vi "main_FP.vi"() -> ()   [LabVIEW 2011]
uses:
  global.vi
  <vilib>/Instr/_visa.llb/VISA Configure Serial Port (Instr).vi
panel:
  out "RN2483 Connected":bool caption="Connected"
  in  "Tab Control 2":T1(tab)
  out "Receiving":bool
  out "Signal Noise Ratio":string="0"
  out "Packet number":i32
  in  "Stop_reception":bool
  in  "Start_reception":bool
  in  "reception_list":i32(listbox)
  out "reception Graph":dbl[](graph)
  out "Transmitting":bool
  in  "delay (ms)":u32=2000 max=65535 step=1
  in  "tx_timestamp":bool caption="Add timestamp"
  in  "tx_packetnum":bool caption="Add packet number"
  in  "Message":string="0"
  out "TX Packet number":i32 caption="Packet number"
  in  "Stop_transmission":bool
  in  "Start_transmission":bool caption="Start_reception"
  in  "transmission_list":i32(listbox)
  in  "Bandwidth":string(combo)="125"
  in  "CRC":bool
  in  "Preamble length":u32=8 max=65535 step=1
  in  "Frequency":u32=57600 max=65535 step=1
  in  "Bitrate":u32=50000 max=65535 step=1
  in  "Freq deviation":u32=57600 max=65535 step=1
  in  "RX signal bw":string(combo)
  in  "Freq correct":string(combo)
  in  "Spreading factor":string(combo)
  in  "Power":string(combo)
  in  "Radio mode":string(combo)
  out "EUI address":string="\r\n"
  out "Voltage":string="\r\n"
  out "Version":string="0004A30B001A5EB1\r\n"
  in  "Save_changes":bool
  in  "Cancel_changes":bool
  out "error":bool
  in  "Discover device":bool=TRUE
  in  "Timeout (ms)":u32=10000
  in  "Port":refnum<visa-resource-name>="COM1"
  in  "Parity":u16(ring) items=["None", "Odd", "Even", "Mark", "Space"]
  in  "Stop bits":u16(ring)=10 items=["1.0"=10, "1.5"=15, "2.0"=20]
  in  "Baud rate":u32=57600
  in  "Data bits":u16=8
  # "Reception mode"
  # "Transmission mode"
  # "Device info"
  # "Device config"
  # "Serial port"
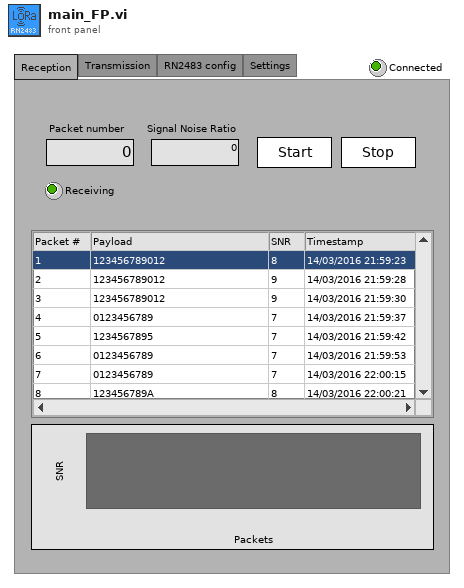
[diagram p1: front panel]
types:
  T1 = enum32{"Reception", "Transmission", "RN2483 config", "Settings"}
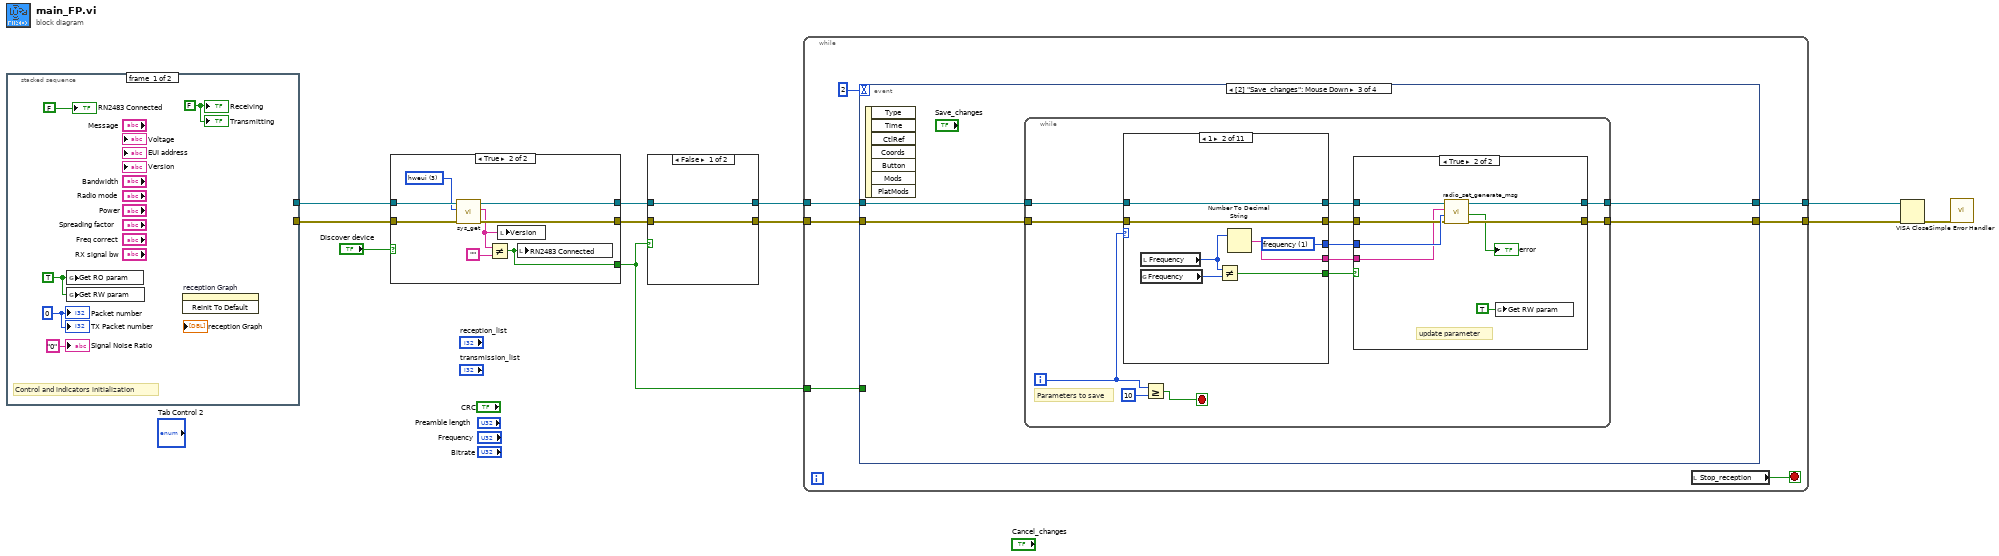
[diagram p0: block diagram]
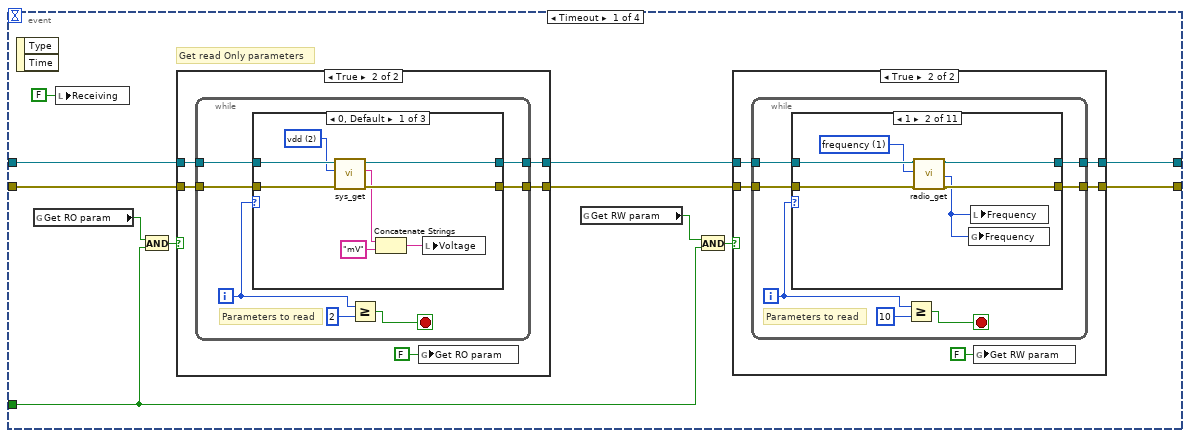
[diagram p2: hidden frame]
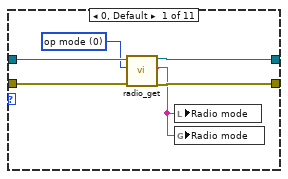
[diagram p4: hidden frame]
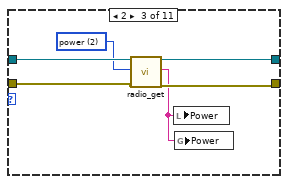
[diagram p5: hidden frame]
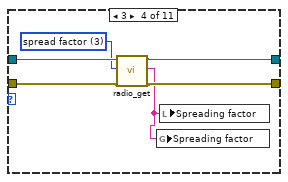
[diagram p6: hidden frame]
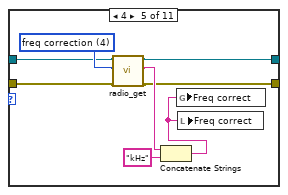
[diagram p7: hidden frame]
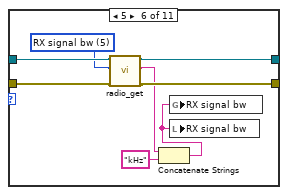
[diagram p8: hidden frame]
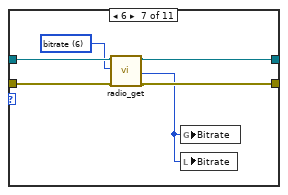
[diagram p9: hidden frame]
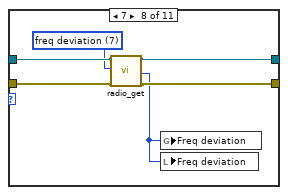
[diagram p10: hidden frame]
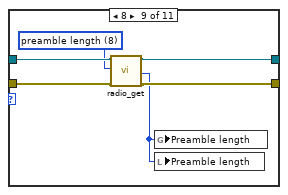
[diagram p11: hidden frame]
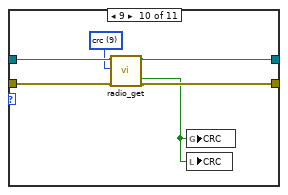
[diagram p12: hidden frame]
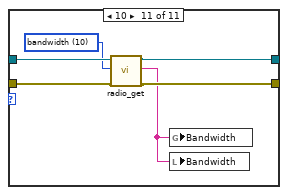
[diagram p13: hidden frame]
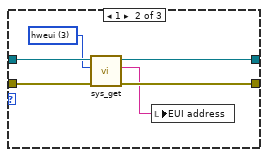
[diagram p15: hidden frame]
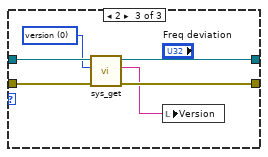
[diagram p16: hidden frame]
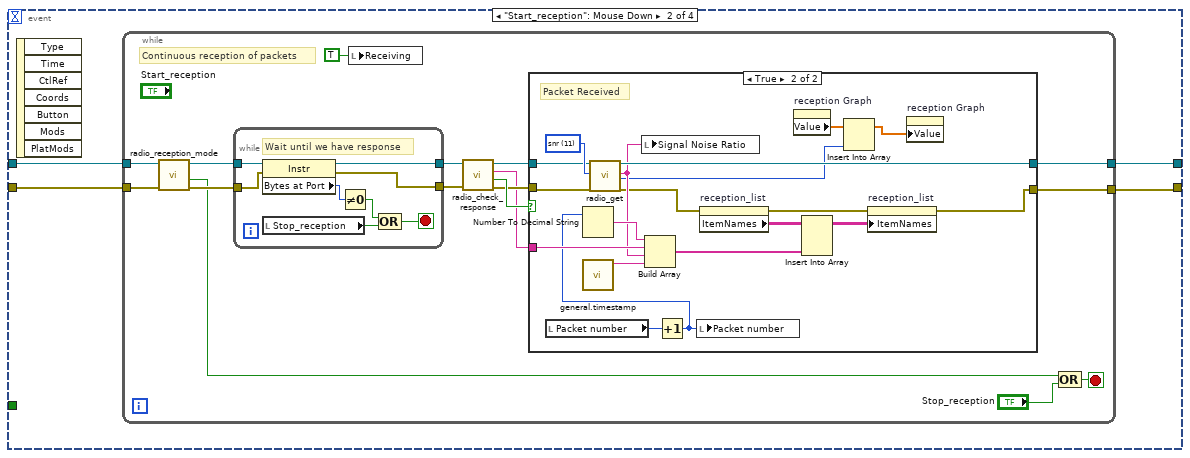
[diagram p17: hidden frame]
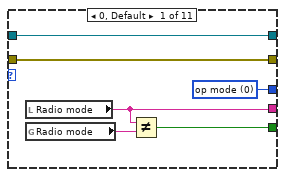
[diagram p20: hidden frame]
diagram:
  n1 = stacked-sequence {
    tunnel: [_ w19] -> w10
    tunnel: [_ w18] -> w9
    frame #0 {
      w12 = FALSE ("Receiving")
      w13 = 0 ("Packet number")
      w15 = TRUE ("Get RO param")
      # "Control and indicators initialization"
      n2 = global write "global.vi" "Get RO param"(w15) -> ()
      n3 = global write "global.vi" "Get RW param"(w15) -> ()
      n4 = invoke on="reception Graph" class="WFGraph (strict)" method="Reinit To Default"() -> ()  [unwired: 3 in, 3 out]
      "RN2483 Connected" <- FALSE ("RN2483 Connected")
      "Packet number" <- w13
      "Signal Noise Ratio" <- "0" ("Signal Noise Ratio")
      "Receiving" <- w12
      "TX Packet number" <- w13
      "Transmitting" <- w12
    }
    frame #1 {
      w22 = u16 0 items=["None", "XON/XOFF", "RTS/CTS", "DTR/DSR"] ("Flow control")
      # "Configure Serial port (baud rate, data bits, parity, stop bits and flow control)."
      n5 = call-poly "VISA Configure Serial Port"("VISA resource name"="Port", "timeout (10sec)"="Timeout (ms)", "baud rate (9600)"="Baud rate", "data bits (8)"="Data bits", "parity (0:none)"="Parity", "stop bits (10: 1 bit)"="Stop bits", "flow control (0:none)"=w22) -> ("VISA resource name out"=w19:refnum<visa-resource-name>, "error out"=w18:errorcluster)  [unwired: 2 in, 5 out]
    }
  }
  n6 = case shown="True" "Discover device" {
    tunnel: [w28 w34] -> w3
    tunnel: w10 -> [w27 w36]
    tunnel: w9 -> [w28 w35]
    tunnel: [w27 w33] -> w4
    tunnel: [FALSE w30] -> w5
    frame False {
    }
    frame True {
      w32 = u16 3 items=["version", "nvm", "vdd", "hweui"] ("Sys get command")
      n7 = call "sys_get.vi"("error in"=w35, "Sys get command"=w32, "VISA in"=w36) -> ("error out"=w34:errorcluster, "response"=w29:string, "VISA out"=w33:refnum<visa-resource-name>)  [unwired: 6 in]
      n8 = Not Equal?(x=w29, y="") -> (x != y?=w30:bool)
      n9 = local write "Version"(w29) -> ()
      n10 = local write "RN2483 Connected"(w30) -> ()
    }
  }
  n11 = case shown="False" w5 {
    tunnel: w4 -> [w38 w42]
    tunnel: w3 -> [w37 w41]
    tunnel: [w38 w40] -> w2
    tunnel: [w37 w39] -> w1
    frame False {
    }
    frame True {
      n12 = call "mac_pause.vi"("error in"=w41, "VISA in"=w42) -> ("error out"=w39:errorcluster, "VISA out"=w40:refnum<visa-resource-name>)  [unwired: 7 in, 1 out]
    }
  }
  n13 = while {
    tunnel: [w49] -> w7
    tunnel: [w48] -> w6
    tunnel: w5 -> [w46]
    tunnel: w2 -> [w45]
    tunnel: w1 -> [w44]
    stop <- w43 stop-if-true
    n14 = event shown="[2] \"Save_changes\": Mouse Down" {
      selector: _ -> [_ _ _ _]
      dyn-events: _ -> [_ _ _ _]
      timeout: 2 -> [_ _ _ _]
      tunnel: [w54 w181 w230 w329] -> w49
      tunnel: [w53 w180 w229 w328] -> w48
      tunnel: w46 -> [w52 _ _ _]
      tunnel: w45 -> [w61 w183 w232 w331]
      tunnel: w44 -> [w60 w182 w231 w330]
      event Timeout {
        # "Get read Only parameters"
        n15 = event-data() -> ()  [unwired: 1 in, 2 out]
        n16 = global read "global.vi" "Get RO param"() -> (w58:bool)
        n17 = local write "Receiving"(FALSE ("Receiving")) -> ()
        n18 = And(x=w58, y=w52) -> (x .and. y?=w59:bool)
        n19 = case shown="True" w59 {
          tunnel: w61 -> [w147 w152]
          tunnel: w60 -> [w146 w151]
          tunnel: [w147 w150] -> w56
          tunnel: [w146 w149] -> w55
          frame False {
            # "Don't read RN2483 parameters"
          }
          frame True {
            n20 = while {
              tunnel: w152 -> [w159]
              tunnel: w151 -> [w158]
              tunnel: [w157] -> w150
              tunnel: [w156] -> w149
              i -> [w153]
              stop <- w154 stop-if-true
              # "Parameters to read"
              n21 = case shown="0, Default" w153 {
                tunnel: w159 -> [w167 w173 w179]
                tunnel: w158 -> [w166 w172 w178]
                tunnel: [w165 w171 w177] -> w157
                tunnel: [w164 w170 w176] -> w156
                frame 0, Default {
                  w163 = u16 2 items=["version", "nvm", "vdd", "hweui"] ("Sys get command")
                  n22 = call "sys_get.vi"("error in"=w166, "Sys get command"=w163, "VISA in"=w167) -> ("error out"=w164:errorcluster, "response"=w161:string, "VISA out"=w165:refnum<visa-resource-name>)  [unwired: 6 in]
                  n23 = Concatenate Strings(w161, "mV" ("string")) -> (w160:string)
                  n24 = local write "Voltage"(w160) -> ()
                }
                frame 1 {
                  w169 = u16 3 items=["version", "nvm", "vdd", "hweui"] ("Sys get command")
                  n25 = call "sys_get.vi"("error in"=w172, "Sys get command"=w169, "VISA in"=w173) -> ("error out"=w170:errorcluster, "response"=w168:string, "VISA out"=w171:refnum<visa-resource-name>)  [unwired: 6 in]
                  n26 = local write "EUI address"(w168) -> ()
                }
                frame 2 {
                  w175 = u16 0 items=["version", "nvm", "vdd", "hweui"] ("Sys get command")
                  n27 = call "sys_get.vi"("error in"=w178, "Sys get command"=w175, "VISA in"=w179) -> ("error out"=w176:errorcluster, "response"=w174:string, "VISA out"=w177:refnum<visa-resource-name>)  [unwired: 6 in]
                  n28 = local write "Version"(w174) -> ()
                }
              }
              n29 = Greater Or Equal?(x=w153, y=2) -> (x >= y?=w154:bool)
            }
            n30 = global write "global.vi" "Get RO param"(FALSE ("Get RO param")) -> ()
          }
        }
        n31 = global read "global.vi" "Get RW param"() -> (w51:bool)
        n32 = And(x=w51, y=w52) -> (x .and. y?=w57:bool)
        n33 = case shown="True" w57 {
          tunnel: w56 -> [w63 w68]
          tunnel: w55 -> [w62 w67]
          tunnel: [w63 w66] -> w54
          tunnel: [w62 w65] -> w53
          frame False {
            # "Don't read RN2483 parameters"
          }
          frame True {
            n34 = while {
              tunnel: w68 -> [w75]
              tunnel: w67 -> [w74]
              tunnel: [w73] -> w66
              tunnel: [w72] -> w65
              i -> [w69]
              stop <- w70 stop-if-true
              # "Parameters to read"
              n35 = case shown="1" w69 {
                tunnel: w75 -> [w81 w86 w93 w98 w101 w110 w120 w126 w132 w138 w144]
                tunnel: w74 -> [w79 w87 w92 w99 w103 w114 w121 w127 w133 w139 w145]
                tunnel: [w78 w84 w90 w97 w106 w112 w118 w124 w130 w136 w143] -> w73
                tunnel: [w77 w83 w89 w96 w104 w113 w117 w123 w129 w135 w142] -> w72
                frame 0, Default {
                  w80 = u16 0 items=["op mode", "frequency", "power", "spread factor"] ("Radio get command")
                  n36 = call "radio_get.vi"("VISA in"=w81, "Radio get command"=w80, "error in"=w79) -> ("VISA out"=w78:refnum<visa-resource-name>, "response"=w76:string, "error out"=w77:errorcluster)  [unwired: 12 in, 2 out]
                  n37 = local write "Radio mode"(w76) -> ()
                  n38 = global write "global.vi" "Radio mode"(w76) -> ()
                }
                frame 1 {
                  w85 = u16 1 items=["op mode", "frequency", "power", "spread factor"] ("Radio get command")
                  n39 = call "radio_get.vi"("VISA in"=w86, "Radio get command"=w85, "error in"=w87) -> ("VISA out"=w84:refnum<visa-resource-name>, "Num out"=w82:u32, "error out"=w83:errorcluster)  [unwired: 12 in, 2 out]
                  n40 = global write "global.vi" "Frequency"(w82) -> ()
                  n41 = local write "Frequency"(w82) -> ()
                }
                frame 2 {
                  w91 = u16 2 items=["op mode", "frequency", "power", "spread factor"] ("Radio get command")
                  n42 = call "radio_get.vi"("VISA in"=w93, "Radio get command"=w91, "error in"=w92) -> ("VISA out"=w90:refnum<visa-resource-name>, "response"=w88:string, "error out"=w89:errorcluster)  [unwired: 12 in, 2 out]
                  n43 = local write "Power"(w88) -> ()
                  n44 = global write "global.vi" "Power"(w88) -> ()
                }
                frame 3 {
                  w95 = u16 3 items=["op mode", "frequency", "power", "spread factor"] ("Radio get command")
                  n45 = call "radio_get.vi"("VISA in"=w98, "Radio get command"=w95, "error in"=w99) -> ("VISA out"=w97:refnum<visa-resource-name>, "response"=w94:string, "error out"=w96:errorcluster)  [unwired: 12 in, 2 out]
                  n46 = global write "global.vi" "Spreading factor"(w94) -> ()
                  n47 = local write "Spreading factor"(w94) -> ()
                }
                frame 4 {
                  w102 = u16 4 items=["op mode", "frequency", "power", "spread factor", "freq correction", "RX signal bw"] ("Radio get command")
                  n48 = call "radio_get.vi"("VISA in"=w101, "Radio get command"=w102, "error in"=w103) -> ("VISA out"=w106:refnum<visa-resource-name>, "response"=w105:string, "error out"=w104:errorcluster)  [unwired: 12 in, 2 out]
                  n49 = Concatenate Strings(w105, "kHz" ("string")) -> (w100:string)
                  n50 = global write "global.vi" "Freq correct"(w100) -> ()
                  n51 = local write "Freq correct"(w100) -> ()
                }
                frame 5 {
                  w109 = u16 5 items=["op mode", "frequency", "power", "spread factor", "freq correction", "RX signal bw"] ("Radio get command")
                  n52 = call "radio_get.vi"("VISA in"=w110, "Radio get command"=w109, "error in"=w114) -> ("VISA out"=w112:refnum<visa-resource-name>, "response"=w111:string, "error out"=w113:errorcluster)  [unwired: 12 in, 2 out]
                  n53 = Concatenate Strings(w111, "kHz" ("string")) -> (w108:string)
                  n54 = global write "global.vi" "RX signal bw"(w108) -> ()
                  n55 = local write "RX signal bw"(w108) -> ()
                }
                frame 6 {
                  w119 = u16 6 items=["op mode", "frequency", "power", "spread factor", "freq correction", "RX signal bw", "bitrate", "freq deviation", "preamble length", "crc"] ("Radio get command")
                  n56 = call "radio_get.vi"("VISA in"=w120, "Radio get command"=w119, "error in"=w121) -> ("VISA out"=w118:refnum<visa-resource-name>, "Num out"=w116:u32, "error out"=w117:errorcluster)  [unwired: 12 in, 2 out]
                  n57 = global write "global.vi" "Bitrate"(w116) -> ()
                  n58 = local write "Bitrate"(w116) -> ()
                }
                frame 7 {
                  w125 = u16 7 items=["op mode", "frequency", "power", "spread factor", "freq correction", "RX signal bw", "bitrate", "freq deviation", "preamble length", "crc"] ("Radio get command")
                  n59 = call "radio_get.vi"("VISA in"=w126, "Radio get command"=w125, "error in"=w127) -> ("VISA out"=w124:refnum<visa-resource-name>, "Num out"=w122:u32, "error out"=w123:errorcluster)  [unwired: 12 in, 2 out]
                  n60 = global write "global.vi" "Freq deviation"(w122) -> ()
                  n61 = local write "Freq deviation"(w122) -> ()
                }
                frame 8 {
                  w131 = u16 8 items=["op mode", "frequency", "power", "spread factor", "freq correction", "RX signal bw", "bitrate", "freq deviation", "preamble length", "crc"] ("Radio get command")
                  n62 = call "radio_get.vi"("VISA in"=w132, "Radio get command"=w131, "error in"=w133) -> ("VISA out"=w130:refnum<visa-resource-name>, "Num out"=w128:u32, "error out"=w129:errorcluster)  [unwired: 12 in, 2 out]
                  n63 = global write "global.vi" "Preamble length"(w128) -> ()
                  n64 = local write "Preamble length"(w128) -> ()
                }
                frame 9 {
                  w137 = u16 9 items=["op mode", "frequency", "power", "spread factor", "freq correction", "RX signal bw", "bitrate", "freq deviation", "preamble length", "crc"] ("Radio get command")
                  n65 = call "radio_get.vi"("VISA in"=w138, "Radio get command"=w137, "error in"=w139) -> ("VISA out"=w136:refnum<visa-resource-name>, "Bool out"=w134:bool, "error out"=w135:errorcluster)  [unwired: 12 in, 2 out]
                  n66 = global write "global.vi" "CRC"(w134) -> ()
                  n67 = local write "CRC"(w134) -> ()
                }
                frame 10 {
                  w141 = u16 10 items=["op mode", "frequency", "power", "spread factor", "freq correction", "RX signal bw", "bitrate", "freq deviation", "preamble length", "crc", "bandwidth"] ("Radio get command")
                  n68 = call "radio_get.vi"("VISA in"=w144, "Radio get command"=w141, "error in"=w145) -> ("VISA out"=w143:refnum<visa-resource-name>, "response"=w140:string, "error out"=w142:errorcluster)  [unwired: 12 in, 2 out]
                  n69 = global write "global.vi" "Bandwidth"(w140) -> ()
                  n70 = local write "Bandwidth"(w140) -> ()
                }
              }
              n71 = Greater Or Equal?(x=w69, y=10) -> (x >= y?=w70:bool)
            }
            n72 = global write "global.vi" "Get RW param"(FALSE ("Get RO param")) -> ()
          }
        }
      }
      event "Start_reception": Mouse Down {
        n73 = event-data() -> ()  [unwired: 1 in, 7 out]
        n74 = while {
          tunnel: w183 -> [w198]
          tunnel: w182 -> [w199]
          tunnel: [w187] -> w181
          tunnel: [w186] -> w180
          stop <- w197 stop-if-true
          # "Continuous reception of packets"
          n75 = call "radio_reception_mode.vi"("error in"=w199, "VISA in"=w198) -> ("error out"=w194:errorcluster, "error"=w184:bool, "VISA out"=w195:refnum<visa-resource-name>)  [unwired: 7 in]
          n76 = while {
            tunnel: w195 -> [w228]
            tunnel: w194 -> [w227]
            tunnel: [w226] -> w192
            tunnel: [w225] -> w193
            stop <- w221 stop-if-true
            # "Wait until we have response"
            n77 = property class="Instr"(reference=w228, error in=w227) -> (reference out=w226:refnum<visa-resource-name>, error out=w225:errorcluster, "Bytes at Port"=w224:u32)
            n78 = local read "Stop_reception"() -> (w222:bool)
            n79 = Not Equal To 0?(x=w224) -> (x != 0?=w223:bool)
            n80 = Compound Arithmetic op=OR(w223, w222) -> (w221:bool)
          }
          n81 = local write "Receiving"(TRUE ("Receiving")) -> ()
          n82 = call "radio_check_response.vi"("error in"=w193, "VISA in"=w192) -> ("error out"=w190:errorcluster, "ok"=w191:bool, "read buffer"=w188:string, "VISA out"=w189:refnum<visa-resource-name>)  [unwired: 6 in]
          n83 = case shown="True" w191 {
            tunnel: w190 -> [w200 w214]
            tunnel: w189 -> [w201 w215]
            tunnel: w188 -> [_ w217]
            tunnel: [w200 w202] -> w186
            tunnel: [w201 w213] -> w187
            frame False {
            }
            frame True {
              w216 = u16 11 items=["op mode", "frequency", "power", "spread factor", "freq correction", "RX signal bw", "bitrate", "freq deviation", "preamble length", "crc", "bandwidth", "snr"] ("Radio get command")
              # "Packet Received"
              n84 = local read "Packet number"() -> (w220:i32)
              n85 = call "general.timestamp.vi"() -> ("timestamp"=w212:string)  [unwired: 11 in]
              n86 = call "radio_get.vi"("VISA in"=w215, "Radio get command"=w216, "error in"=w214) -> ("VISA out"=w213:refnum<visa-resource-name>, "response"=w208:string, "Num out"=w206:u32, "error out"=w204:errorcluster)  [unwired: 12 in, 1 out]
              n87 = local write "Signal Noise Ratio"(w208) -> ()
              n88 = Increment(x=w220) -> (x+1=w209:i32)
              n89 = Number To Decimal String(number=w209) -> (decimal integer string=w218:string)  [unwired: 1 in]
              n90 = Build Array(w218, w217, w208, w212) -> (w211:string[])
              n91 = local write "Packet number"(w209) -> ()
              n92 = property on="reception_list" class="MCListbox (strict)"(error in=w204) -> (error out=w203:errorcluster, "ItemNames"=w219:string[][])  [unwired: 1 in, 1 out]
              n93 = property on="reception Graph" class="WFGraph (strict)"() -> ("Value"=w207:dbl[])  [unwired: 2 in, 2 out]
              n94 = Insert Into Array(array=w219, new element=w211) -> (w210:string[][])  [unwired: 2 in]
              n95 = Insert Into Array(array=w207, new element=w206) -> (w205:dbl[])  [unwired: 1 in]
              n96 = property on="reception_list" class="MCListbox (strict)"(error in=w203, "ItemNames"=w210) -> (error out=w202:errorcluster)  [unwired: 1 in, 1 out]
              n97 = property on="reception Graph" class="WFGraph (strict)"("Value"=w205) -> ()  [unwired: 2 in, 2 out]
            }
          }
          n98 = Compound Arithmetic op=OR(w184, "Stop_reception") -> (w197:bool)
        }
      }
      event "Save_changes": Mouse Down {
        n99 = event-data() -> ()  [unwired: 1 in, 7 out]
        n100 = while {
          tunnel: w232 -> [w244]
          tunnel: w231 -> [w243]
          tunnel: [w237] -> w230
          tunnel: [w236] -> w229
          i -> [w240]
          stop <- w241 stop-if-true
          # "Parameters to save"
          n101 = case shown="1" w240 {
            tunnel: w244 -> [w257 w262 w269 w275 w281 w287 w293 w300 w307 w319 w323]
            tunnel: w243 -> [w256 w261 w268 w274 w280 w286 w292 w299 w306 w318 w322]
            tunnel: [w257 w262 w269 w275 w281 w287 w293 w300 w307 w319 w323] -> w239
            tunnel: [w256 w261 w268 w274 w280 w286 w292 w299 w306 w318 w322] -> w238
            tunnel: [w259 w266 w272 w278 w284 w290 w297 w304 w311 w317 w326] -> w235
            tunnel: [w255 w263 w270 w276 w282 w288 w294 w301 w308 w313 w324] -> w234
            tunnel: [w258 w265 w271 w277 w283 w289 w296 w303 w310 w320 w325] -> w233
            frame 0, Default {
              w258 = u16 0 items=["op mode", "frequency", "power", "spread factor", "freq correction", "RX signal bw", "bitrate", "freq deviation", "preamble length", "crc", "bandwidth"] ("Radio get command")
              n102 = local read "Radio mode"() -> (w255:string)
              n103 = global read "global.vi" "Radio mode"() -> (w260:string)
              n104 = Not Equal?(x=w255, y=w260) -> (x != y?=w259:bool)
            }
            frame 1 {
              w265 = u16 1 items=["op mode", "frequency", "power", "spread factor", "freq correction", "RX signal bw", "bitrate", "freq deviation", "preamble length", "crc", "bandwidth"] ("Radio get command")
              n105 = global read "global.vi" "Frequency"() -> (w267:u32)
              n106 = local read "Frequency"() -> (w264:u32)
              n107 = Not Equal?(x=w264, y=w267) -> (x != y?=w266:bool)
              n108 = Number To Decimal String(number=w264) -> (decimal integer string=w263:string)  [unwired: 1 in]
            }
            frame 2 {
              w271 = u16 2 items=["op mode", "frequency", "power", "spread factor", "freq correction", "RX signal bw", "bitrate", "freq deviation", "preamble length", "crc", "bandwidth"] ("Radio get command")
              n109 = local read "Power"() -> (w270:string)
              n110 = global read "global.vi" "Power"() -> (w273:string)
              n111 = Not Equal?(x=w270, y=w273) -> (x != y?=w272:bool)
            }
            frame 3 {
              w277 = u16 3 items=["op mode", "frequency", "power", "spread factor", "freq correction", "RX signal bw", "bitrate", "freq deviation", "preamble length", "crc", "bandwidth"] ("Radio get command")
              n112 = local read "Spreading factor"() -> (w276:string)
              n113 = global read "global.vi" "Spreading factor"() -> (w279:string)
              n114 = Not Equal?(x=w276, y=w279) -> (x != y?=w278:bool)
            }
            frame 4 {
              w283 = u16 4 items=["op mode", "frequency", "power", "spread factor", "freq correction", "RX signal bw", "bitrate", "freq deviation", "preamble length", "crc", "bandwidth"] ("Radio get command")
              n115 = local read "Freq correct"() -> (w282:string)
              n116 = global read "global.vi" "Freq correct"() -> (w285:string)
              n117 = Not Equal?(x=w282, y=w285) -> (x != y?=w284:bool)
            }
            frame 5 {
              w289 = u16 5 items=["op mode", "frequency", "power", "spread factor", "freq correction", "RX signal bw", "bitrate", "freq deviation", "preamble length", "crc", "bandwidth"] ("Radio get command")
              n118 = local read "RX signal bw"() -> (w288:string)
              n119 = global read "global.vi" "RX signal bw"() -> (w291:string)
              n120 = Not Equal?(x=w288, y=w291) -> (x != y?=w290:bool)
            }
            frame 6 {
              w296 = u16 6 items=["op mode", "frequency", "power", "spread factor", "freq correction", "RX signal bw", "bitrate", "freq deviation", "preamble length", "crc", "bandwidth"] ("Radio get command")
              n121 = local read "Bitrate"() -> (w295:u32)
              n122 = global read "global.vi" "Bitrate"() -> (w298:u32)
              n123 = Not Equal?(x=w295, y=w298) -> (x != y?=w297:bool)
              n124 = Number To Decimal String(number=w295) -> (decimal integer string=w294:string)  [unwired: 1 in]
            }
            frame 7 {
              w303 = u16 7 items=["op mode", "frequency", "power", "spread factor", "freq correction", "RX signal bw", "bitrate", "freq deviation", "preamble length", "crc", "bandwidth"] ("Radio get command")
              n125 = global read "global.vi" "Freq deviation"() -> (w305:u32)
              n126 = local read "Freq deviation"() -> (w302:u32)
              n127 = Not Equal?(x=w302, y=w305) -> (x != y?=w304:bool)
              n128 = Number To Decimal String(number=w302) -> (decimal integer string=w301:string)  [unwired: 1 in]
            }
            frame 8 {
              w310 = u16 8 items=["op mode", "frequency", "power", "spread factor", "freq correction", "RX signal bw", "bitrate", "freq deviation", "preamble length", "crc", "bandwidth"] ("Radio get command")
              n129 = global read "global.vi" "Preamble length"() -> (w312:u32)
              n130 = local read "Preamble length"() -> (w309:u32)
              n131 = Not Equal?(x=w309, y=w312) -> (x != y?=w311:bool)
              n132 = Number To Decimal String(number=w309) -> (decimal integer string=w308:string)  [unwired: 1 in]
            }
            frame 9 {
              w320 = u16 8 items=["op mode", "frequency", "power", "spread factor", "freq correction", "RX signal bw", "bitrate", "freq deviation", "preamble length", "crc", "bandwidth"] ("Radio get command")
              n133 = global read "global.vi" "CRC"() -> (w321:bool)
              n134 = local read "CRC"() -> (w316:bool)
              n135 = Not Equal?(x=w316, y=w321) -> (x != y?=w317:bool)
              n136 = Select(t="on", s=w316, f="off") -> (s? t:f=w313:string)
            }
            frame 10 {
              w325 = u16 10 items=["op mode", "frequency", "power", "spread factor", "freq correction", "RX signal bw", "bitrate", "freq deviation", "preamble length", "crc", "bandwidth"] ("Radio get command")
              n137 = local read "Bandwidth"() -> (w324:string)
              n138 = global read "global.vi" "Bandwidth"() -> (w327:string)
              n139 = Not Equal?(x=w324, y=w327) -> (x != y?=w326:bool)
            }
          }
          n140 = Greater Or Equal?(x=w240, y=10) -> (x >= y?=w241:bool)
          n141 = case shown="True" w235 {
            tunnel: [w246 w251] -> w237
            tunnel: [w245 w250] -> w236
            tunnel: w239 -> [w246 w253]
            tunnel: w238 -> [w245 w252]
            tunnel: w234 -> [_ w249]
            tunnel: w233 -> [_ w254]
            frame False {
              # "Parameter not changed,\ndo nothing"
            }
            frame True {
              # "update parameter"
              n142 = call "radio_set_generate_msg.vi"("error in"=w252, "Radio command"=w254, "input parameter"=w249, "VISA in"=w253) -> ("error out"=w250:errorcluster, "error"=→"error":bool, "VISA out"=w251:refnum<visa-resource-name>)  [unwired: 4 in, 1 out]
              n143 = global write "global.vi" "Get RW param"(TRUE ("Get RW param")) -> ()
            }
          }
        }
      }
      event "Start_transmission": Mouse Down {
        n144 = event-data() -> ()  [unwired: 1 in, 7 out]
        n145 = while {
          tunnel: w331 -> [w358]
          tunnel: w330 -> [w357]
          tunnel: [w362] -> w329
          tunnel: [w361] -> w328
          i -> [w333]
          stop <- w363 stop-if-true
          # "Continuous reception of packets"
          n146 = local read "Message"() -> (w354:string)
          n147 = call "general.timestamp.vi"() -> ("timestamp"=w346:string)  [unwired: 11 in]
          n148 = Number To Decimal String(number=w333) -> (decimal integer string=w348:string)  [unwired: 1 in]
          n149 = Concatenate Strings(w348, "_" ("element")) -> (w349:string)
          n150 = Concatenate Strings(w354, "_" ("element")) -> (w352:string)
          n151 = Empty String/Path?(string/path=w354) -> (empty?=w356:bool)
          n152 = Concatenate Strings(w346, "_" ("element")) -> (w343:string)
          n153 = Select(t=w349, s="tx_packetnum", f="") -> (s? t:f=w341:string)
          n154 = Select(t="", s=w356, f=w352) -> (s? t:f=w340:string)
          n155 = Select(t=w343, s="tx_timestamp", f="") -> (s? t:f=w339:string)
          n156 = Concatenate Strings(w340, w341, w339) -> (w335:string)
          n157 = local write "Transmitting"(TRUE ("Receiving")) -> ()
          n158 = call "general.ascii2hex.vi"("Ascii input Message"=w335) -> ("Hex output Message"=w334:string)  [unwired: 10 in]
          n159 = local write "TX Packet number"(w333) -> ()
          n160 = call "radio_transmission_mode.vi"("error in"=w357, "message"=w334, "VISA in"=w358) -> ("error out"=w336:errorcluster, "error"=w338:bool, "VISA out"=w337:refnum<visa-resource-name>)  [unwired: 6 in]
          n161 = case shown="False" w338 {
            tunnel: w336 -> [w364 w375]
            tunnel: w337 -> [w370 w376]
            tunnel: w335 -> [w373 _]
            tunnel: [w368 w375] -> w361
            tunnel: [w370 w376] -> w362
            tunnel: w333 -> [w371 _]
            frame False {
              # "Packet transmitted succesfully"
              n162 = Number To Decimal String(number=w371) -> (decimal integer string=w374:string)  [unwired: 1 in]
              n163 = call "general.timestamp.vi"() -> ("timestamp"=w369:string)  [unwired: 11 in]
              n164 = Build Array(w374, w373, w369) -> (w372:string[])
              n165 = property on="transmission_list" class="MCListbox (strict)"(error in=w364) -> (error out=w365:errorcluster, "ItemNames"=w367:string[][])  [unwired: 1 in, 1 out]
              n166 = Insert Into Array(array=w367, new element=w372) -> (w366:string[][])  [unwired: 2 in]
              n167 = property on="transmission_list" class="MCListbox (strict)"(error in=w365, "ItemNames"=w366) -> (error out=w368:errorcluster)  [unwired: 1 in, 1 out]
            }
            frame True {
            }
          }
          n168 = Compound Arithmetic op=OR(w338, "Stop_transmission") -> (w363:bool)
          n169 = Wait (ms)(milliseconds to wait="delay (ms)") -> ()  [unwired: 1 out]
        }
      }
    }
    n170 = local read "Stop_reception"() -> (w43:bool)
  }
  n171 = VISA Close(VISA resource name=w7, error in (no error)=w6) -> (error out=w8:errorcluster)
  n172 = call <vilib>:"Simple Error Handler.vi"("error in (no error)"=w8) -> ()  [unwired: 1 in, 8 out]
